vi "Measurement.GetProtectedEvents.vi"(8 "error in (no error)":errorcluster, 11 "Measurement in":refnum<class "Measurement.lvclass">) -> (0 "error out":errorcluster, 2 "Protected Events":T1, 3 "Measurement out":refnum<class "Measurement.lvclass">)   [LabVIEW 2017, in "Measurement.lvclass"]
uses:
  Measurement.lvclass
  Typedefs/ProtectedEvents--Cluster.ctl
  Typedefs/ProtectedEvents--Measurement.Begin.ctl
  Typedefs/ProtectedEvents--Measurement.Pause.ctl
  Typedefs/ProtectedEvents--Measurement.End.ctl
  Typedefs/ProtectedEvents--Measurement.Uninitialize.ctl
  Measurement.lvclass/Measurement.ctl
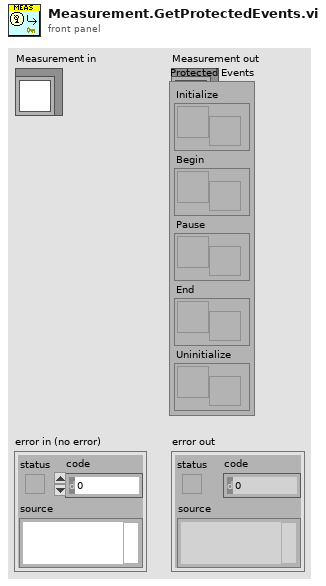
[diagram p1: front panel]
types:
  T1 = typedef "Measurement.lvclass/ProtectedEvents--Cluster.ctl" = cluster{"Initialize":refnum<user-event>, "Begin":refnum<user-event>, "Pause":refnum<user-event>, "End":refnum<user-event>, "Uninitialize":refnum<user-event>}
  T2 = typedef "Measurement.lvclass/PrivateData--Ref.ctl" = refnum<data-value>
  T3 = typedef "Measurement.lvclass/PrivateData--Cluster.ctl" = cluster{"Public Events":T4, "Protected Events":T1}
  T4 = typedef "Measurement.lvclass/PublicEvents--Cluster.ctl" = cluster{"Initialized":refnum<user-event>, "Measured":refnum<user-event>, "Uninitialized":refnum<user-event>}
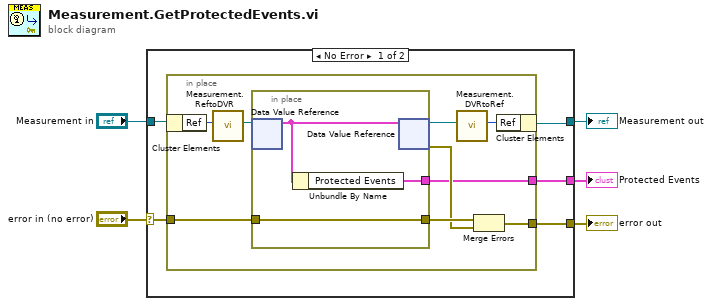
[diagram p0: block diagram]
diagram:
  n1 = case shown="No Error" "error in (no error)" {
    selector: "error in (no error)" -> [w7 w24]
    tunnel: [w6 w24] -> w4
    tunnel: [w9 w23] -> w2
    tunnel: "Measurement in" -> [w10 w23]
    tunnel: [w8 _] -> w1
    frame No Error {
      n2 = in-place {
        in-place-border: w7 -> [w15]
        in-place-border: [w12] -> w6
        in-place-border: [w11] -> w8
        n3 = in-place-cluster #1(w10) -> ("Ref"=w19:u32)
        n4 = call "Measurement.ReftoDVR.vi"("Ref"=w19) -> ("Ref"=w18:T2)  [unwired: 10 in]
        n5 = in-place {
          in-place-border: w15 -> [w21]
          in-place-border: [w21] -> w14
          in-place-border: [w22] -> w11
          n6 = in-place-dvr #2(w18) -> (w20:T3)  [unwired: 1 out]
          n7 = Unbundle By Name(w20) -> ("Protected Events"=w22:T1)
          n8 = in-place-dvr #2(w20) -> (w17:T2, w13:errorcluster)
        }
        n9 = call "Measurement.DVRtoRef.vi"("Ref"=w17) -> ("Ref"=w16:u32)  [unwired: 10 in]
        n10 = Merge Errors(w14, w13) -> (w12:errorcluster)
        n11 = in-place-cluster #1("Ref"=w16) -> (w9:refnum<class "Measurement.lvclass">)
      }
    }
    frame Error {
    }
  }
  "error out" <- w4
  "Measurement out" <- w2
  "Protected Events" <- w1
